vi "IIR Filter (CDB).vi"(2 "init/cont (init:F)":bool, 3 "Forward Coefficients":dbl[](array[numeric]), 4 "Reverse Coefficients":dbl[](array[numeric]), 5 "X":cdb[](array[numeric])) -> (0 "error":i32, 1 "Filtered X":cdb[](array[numeric]))   [LabVIEW 2020, in "NI_AALBase.lvlib"]
doc: "Filters the input sequence <B>X</B> using the direct form IIR filter specified by <B>Reverse Coefficients</B> and <B>Forward Coefficients</B>. Wire data to the <B>X</B> input to determine the polymorphic instance to use or manually select the instance."
uses:
  <vilib>/Analysis/NI_AALBase.lvlib
  <resource>/lvanlys.dll
panel:
  # "IIR Filter"
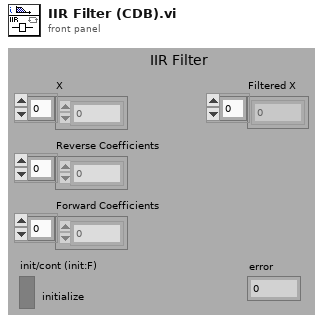
[diagram p1: front panel]
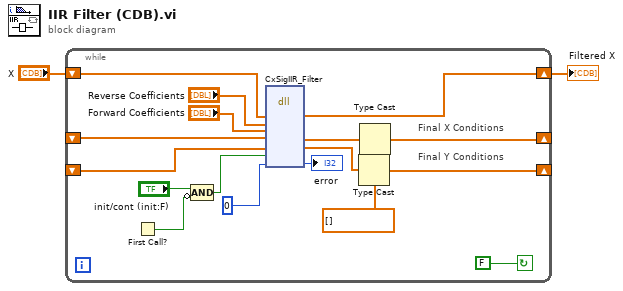
[diagram p0: block diagram]
diagram:
  n1 = while {
    shift-left: _ -> [w10]
    shift-right: [w18] -> _
    shift-left: _ -> [w12]
    shift-right: [w19] -> _
    shift-right: [w3] -> w1
    shift-left: "X" -> [w4]
    stop <- FALSE continue-if-true
    w17 = cdb[] [] ("type for the shift register")
    # "Final Y Conditions"
    # "Final X Conditions"
    n2 = First Call?() -> (First Call?: T/F=w7:bool)
    n3 = Compound Arithmetic op=AND("init/cont (init:F)", invert w7) -> (w5:bool)
    n4 = dll-call lib="e:/builds/penguin/labview/branches/2020/dev/dist/resource/lvanlys.*" fn="CxSigIIR_Filter"("X"=w4, "Reverse Coefficients"="Reverse Coefficients", "Forward Coefficients"="Forward Coefficients", "type for the shift register"=w12, "type for the shift register"=w10, w5, "dsperr"=0) -> ("X"=w3:cdb[], "type for the shift register"=w11:cdb[], "type for the shift register"=w9:cdb[], "dsperr"=→"error":i32)  [unwired: 7 in, 2 out]
    n5 = Type Cast(type=w17, x=w9) -> (*(type *) &x=w18:cdb[])
    n6 = Type Cast(type=w17, x=w11) -> (*(type *) &x=w19:cdb[])
  }
  "Filtered X" <- w1
